vi "single use states FG.vi"(6 "exit in":bool, 8 "state # in":i32, 10 "menu (get)":enum16{"set", "get"}(ring)=enum."get", 11 "substate":T1) -> (0 "first call?":bool, 1 "exit out":bool, 2 "state # out":i32, 3 "substate out":T1)   [LabVIEW 2013]
uses:
  typedefs/singleUseSubstate.ctl
panel:
  # "The All-Powerful Functional Global with all the States (Single Use)"
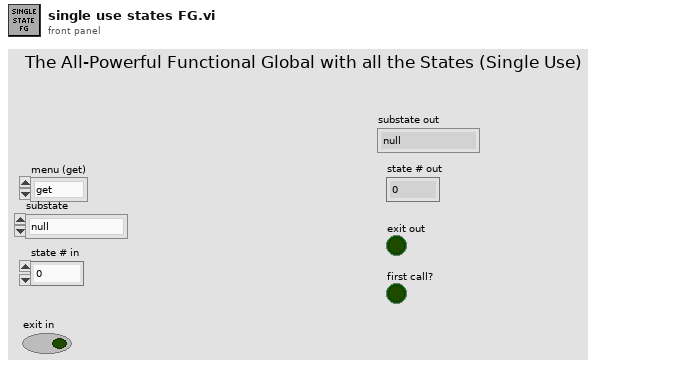
[diagram p1: front panel]
types:
  T1 = typedef "singleUseSubstate.ctl" = enum16{"null", "wait", "shift high", "shift low", "extend shooter", "retract shooter", "close latch", "open latch"}
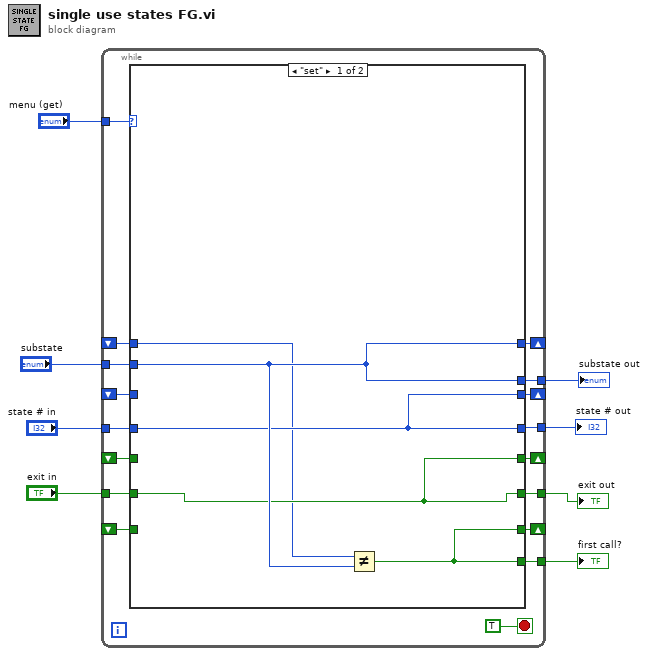
[diagram p0: block diagram]
diagram:
  n1 = while {
    tunnel: "menu (get)" -> [w25]
    shift-right: [w21] -> _
    shift-left: _ -> [w22]
    shift-right: [w20] -> _
    shift-left: _ -> [w23]
    tunnel: "substate" -> [w19]
    tunnel: "state # in" -> [w18]
    tunnel: [w17] -> w1
    tunnel: [w16] -> w6
    shift-right: [w15] -> _
    shift-left: _ -> [w14]
    tunnel: [w13] -> w4
    tunnel: "exit in" -> [w12]
    shift-right: [w11] -> _
    shift-left: _ -> [w10]
    tunnel: [w9] -> w3
    stop <- TRUE stop-if-true
    n2 = case shown="\"set\"" w25 {
      tunnel: w23 -> [_ w33]
      tunnel: w22 -> [w26 w34]
      tunnel: [w30 w34] -> w17
      tunnel: [w30 w34] -> w21
      tunnel: [w29 w33] -> w20
      tunnel: [w29 w33] -> w16
      tunnel: w19 -> [w30 _]
      tunnel: w18 -> [w29 _]
      tunnel: [w28 w32] -> w15
      tunnel: w14 -> [_ w32]
      tunnel: [w28 w32] -> w13
      tunnel: w12 -> [w28 _]
      tunnel: [w27 w31] -> w11
      tunnel: w10 -> [_ w31]
      tunnel: [w27 w31] -> w9
      frame "set" {
        n3 = Not Equal?(x=w26, y=w30) -> (x != y?=w27:bool)
      }
      frame "get", Default {
      }
    }
  }
  "state # out" <- w6
  "exit out" <- w4
  "first call?" <- w3
  "substate out" <- w1
